vi "FID mit Propan Kalibrieren.vi"(6 "Aktionen":T2, 10 "Wert":sgl=1.07, 11 "FID Kal Komponente":T1) -> (2 "Wert":sgl, 3 "FID Kal Komponente":T1)   [LabVIEW 2020, in "ABB-EL3000.lvlib" / "FID.lvlib" / "FID Kalibrierung.lvlib"]
uses:
  FID Kalibrierung.lvlib
  FID Kal Komponente.ctl
  Aktionen FID Kal Komponente.ctl
  <vilib>/Utility/config.llb/Read Key (U32).vi
  <vilib>/Utility/config.llb/Write Key (U32).vi
  <vilib>/Utility/config.llb/NI_LVConfig.lvlib
  Allgemein/allgemeine Sub-VIs.lvlib
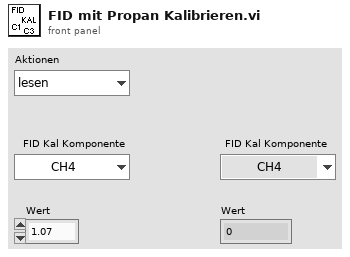
[diagram p1: front panel]
types:
  T1 = typedef "ABB-EL3000.lvlib/FID.lvlib/FID Kalibrierung.lvlib/FID Kal Komponente.ctl" = enum16{"CH4", "C3H8"}
  T2 = typedef "ABB-EL3000.lvlib/FID.lvlib/FID Kalibrierung.lvlib/Aktionen FID Kal Komponente.ctl" = enum16{"lesen", "setzen", "laden", "speichern", "LIN"}
  T3 = typedef "NI_LVConfig.lvlib/Config Data RefNum.ctl" = refnum<k1>
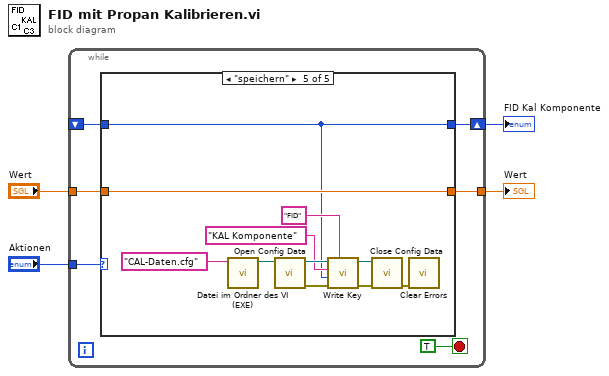
[diagram p0: block diagram]
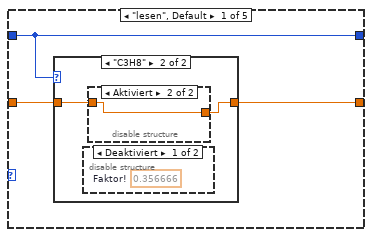
[diagram p2: hidden frame]
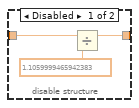
[diagram p4: hidden frame]
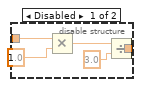
[diagram p5: hidden frame]
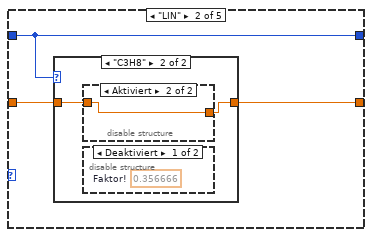
[diagram p7: hidden frame]
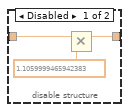
[diagram p9: hidden frame]
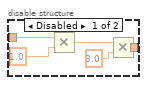
[diagram p10: hidden frame]
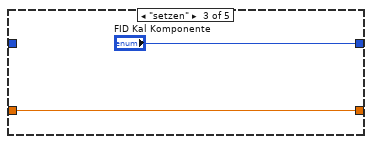
[diagram p12: hidden frame]
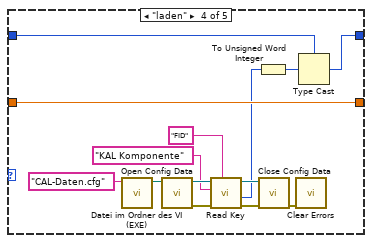
[diagram p13: hidden frame]
diagram:
  n1 = while {
    tunnel: [w10] -> w4
    tunnel: "Wert" -> [w9]
    tunnel: "Aktionen" -> [w8]
    shift-right: [w6] -> w1
    shift-left: _ -> [w5]
    stop <- TRUE stop-if-true
    n2 = case shown="\"speichern\"" w8 {
      tunnel: [w13 w30 w45 w51 w71] -> w10
      tunnel: w9 -> [w12 w29 w45 w51 w71]
      tunnel: [w11 w28 "FID Kal Komponente" w53 w63] -> w6
      tunnel: w5 -> [w11 w28 _ w52 w63]
      frame "lesen", Default {
        n3 = case shown="\"C3H8\"" w11 {
          tunnel: w12 -> [w15 w21]
          tunnel: [w14 w20] -> w13
          frame "CH4", Default {
            n4 = disable-structure shown="Aktiviert" {
              disable-tunnel: w15 -> [w18 w19]
              disable-tunnel: [w17 w19] -> w14
              frame Disabled {
                n5 = Divide(x=w18, y=sgl 1.106) -> (x/y=w17:sgl)
              }
              frame Enabled {
              }
            }
          }
          frame "C3H8" {
            n6 = disable-structure shown="Deaktiviert" {
              frame Disabled {
                (unwired) 0.356666  # Faktor!
              }
              frame Enabled {
              }
            }
            n7 = disable-structure shown="Aktiviert" {
              disable-tunnel: w21 -> [w26 w27]
              disable-tunnel: [w25 w27] -> w20
              frame Disabled {
                n8 = Multiply(x=w26, y=sgl 1.0) -> (x*y=w23:sgl)
                n9 = Divide(x=w23, y=sgl 3.0) -> (x/y=w25:sgl)
              }
              frame Enabled {
              }
            }
          }
        }
      }
      frame "LIN" {
        n10 = case shown="\"C3H8\"" w28 {
          tunnel: w29 -> [w32 w38]
          tunnel: [w31 w37] -> w30
          frame "CH4", Default {
            n11 = disable-structure shown="Aktiviert" {
              disable-tunnel: w32 -> [w35 w36]
              disable-tunnel: [w34 w36] -> w31
              frame Disabled {
                n12 = Multiply(x=w35, y=sgl 1.106) -> (x*y=w34:sgl)
              }
              frame Enabled {
              }
            }
          }
          frame "C3H8" {
            n13 = disable-structure shown="Aktiviert" {
              disable-tunnel: w38 -> [w43 w44]
              disable-tunnel: [w42 w44] -> w37
              frame Disabled {
                n14 = Multiply(x=w43, y=sgl 1.0) -> (x*y=w40:sgl)
                n15 = Multiply(x=w40, y=sgl 3.0) -> (x*y=w42:sgl)
              }
              frame Enabled {
              }
            }
            n16 = disable-structure shown="Deaktiviert" {
              frame Disabled {
                (unwired) 0.356666  # Faktor!
              }
              frame Enabled {
              }
            }
          }
        }
      }
      frame "setzen" {
      }
      frame "laden" {
        n17 = call "Datei im Ordner des VI (EXE).vi"("Dateiname"="CAL-Daten.cfg") -> ("Dateipfad im Ordner des Haupt-VIs"=w47:path)  [unwired: 8 in, 2 out]
        n18 = call <vilib>:"Open Config Data.vi"("configuration file path"=w47) -> ("error out"=w59:errorcluster, "refnum"=w58:T3)  [unwired: 8 in, 1 out]
        n19 = call-poly <vilib>:"Read Key.vi"("section"="FID", "error in (no error)"=w59, "key"="KAL Komponente", "refnum"=w58) -> ("error out"=w56:errorcluster, "value"=w49:u32, "refnum out"=w57:T3)  [unwired: 4 in, 1 out]
        n20 = To Unsigned Word Integer(number=w49) -> (unsigned 16bit integer=w50:u16)
        n21 = call <vilib>:"Close Config Data.vi"("error in (no error)"=w56, "refnum"=w57) -> ("error out"=w60:errorcluster)  [unwired: 1 in, 8 out]
        n22 = call <vilib>:"Clear Errors.vi"("error in (no error)"=w60) -> ()  [unwired: 5 in, 2 out]
        n23 = Type Cast(type=w52, x=w50) -> (*(type *) &x=w53:T1)
      }
      frame "speichern" {
        n24 = call "Datei im Ordner des VI (EXE).vi"("Dateiname"="CAL-Daten.cfg") -> ("Dateipfad im Ordner des Haupt-VIs"=w61:path)  [unwired: 8 in, 2 out]
        n25 = call <vilib>:"Open Config Data.vi"("configuration file path"=w61) -> ("error out"=w70:errorcluster, "refnum"=w69:T3)  [unwired: 8 in, 1 out]
        n26 = call-poly <vilib>:"Write Key.vi"("section"="FID", "error in (no error)"=w70, "value"=w63, "key"="KAL Komponente", "refnum"=w69) -> ("error out"=w67:errorcluster, "refnum out"=w68:T3)  [unwired: 4 in, 1 out]
        n27 = call <vilib>:"Close Config Data.vi"("error in (no error)"=w67, "refnum"=w68) -> ("error out"=w66:errorcluster)  [unwired: 1 in, 8 out]
        n28 = call <vilib>:"Clear Errors.vi"("error in (no error)"=w66) -> ()  [unwired: 5 in, 2 out]
      }
    }
  }
  "Wert" <- w4
  "FID Kal Komponente" <- w1
